vi "clearBuffer.vi"(8 "error in (no error)":errorcluster, 11 "DomeCommunicator in":refnum<class "ATDomeCommunicator.lvclass">) -> (0 "error out":errorcluster, 1 "timeout":bool, 2 "response":string, 3 "DomeCommunicator out":refnum<class "ATDomeCommunicator.lvclass">)   [LabVIEW 2016, in "ATDomeCommunicator.lvclass"]
uses:
  ATDomeCommunicator.lvclass
  home/plotz/lsst_ts/ss_atDome/common_labview_tcpdevice/tcpDevice/tcpDevice.lvclass
  common_labview_tcpdevice/tcpDevice/tcpDevice.lvclass
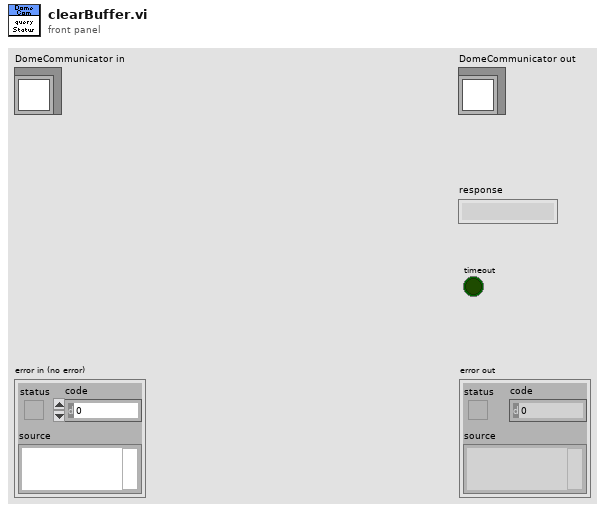
[diagram p1: front panel]
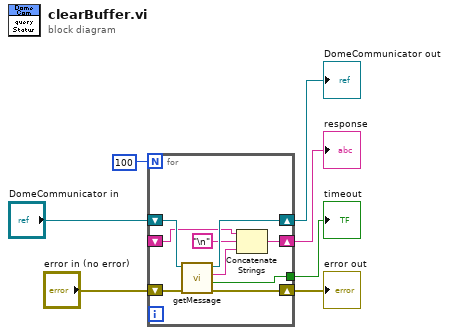
[diagram p0: block diagram]
diagram:
  n1 = for {
    N: 100 -> [_]
    tunnel: [w14] -> w4
    shift-right: [w16] -> w7
    shift-left: "DomeCommunicator in" -> [w13]
    shift-right: [w15] -> w6
    shift-left: "error in (no error)" -> [w12]
    shift-right: [w10] -> w5
    shift-left: _ -> [w9]
    n2 = call "getMessage.vi"("error in (no error)"=w12, "tcpDevice in"=w13) -> ("error out"=w15:errorcluster, "timeout"=w14:bool, "Message"=w11:string, "tcpDevice out"=w16:refnum<class "ATDomeCommunicator.lvclass">)  [unwired: 6 in]
    n3 = Concatenate Strings(w9, "\n", w11) -> (w10:string)
  }
  "error out" <- w6
  "DomeCommunicator out" <- w7
  "response" <- w5
  "timeout" <- w4
